vi "실습 6-2 신호시뮬레이션(이벤트).vi"() -> ()   [LabVIEW 2014]
uses:
  <vilib>/Analysis/NI_AALBase.lvlib
panel:
  in  "정지":bool
  out "웨이브폼 그래프":dbl[](graph)
  in  "열거형":enum16{"사인파", "삼각파", "사각파", "톱니파", "노이즈"}(ring)
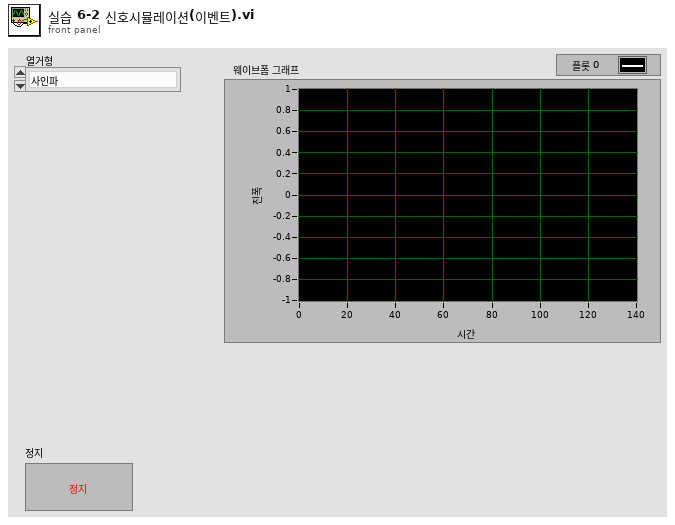
[diagram p1: front panel]
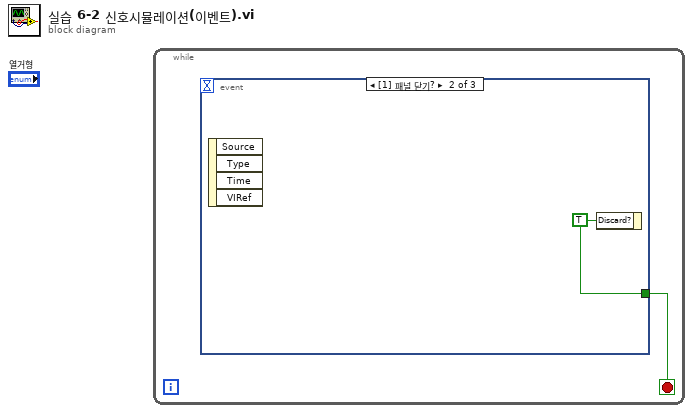
[diagram p0: block diagram]
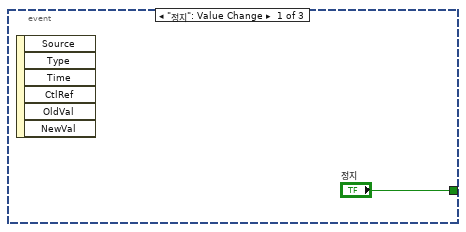
[diagram p2: hidden frame]
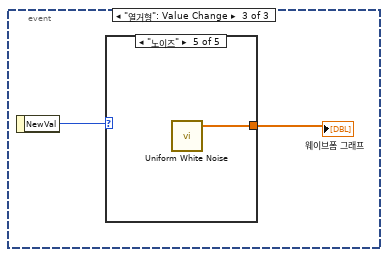
[diagram p3: hidden frame]
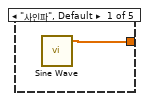
[diagram p4: hidden frame]
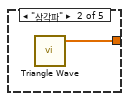
[diagram p5: hidden frame]
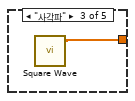
[diagram p6: hidden frame]
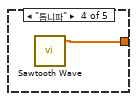
[diagram p7: hidden frame]
diagram:
  n1 = while {
    stop <- w1 stop-if-true
    n2 = event shown="[1] 패널 닫기?" {
      selector: _ -> [_ _ _]
      dyn-events: _ -> [_ _ _]
      timeout: _ -> [_ _ _]
      tunnel: ["정지" w3 _] -> w1
      event "정지": Value Change {
        n3 = event-data() -> ()  [unwired: 1 in, 6 out]
      }
      event Panel Close? {
        w3 = TRUE ("버림?")
        n4 = event-data() -> ()  [unwired: 1 in, 4 out]
        n5 = event-data("Discard?"=w3) -> ()  [unwired: 1 in, 1 out]
      }
      event "열거형": Value Change {
        n6 = event-data() -> ("NewVal"=w5:enum16{"사인파", "삼각파", "사각파", "톱니파", "노이즈"})  [unwired: 1 in]
        n7 = case shown="\"노이즈\"" w5 {
          tunnel: [w6 w7 w8 w9 w10] -> w4
          frame "사인파", Default {
            n8 = call <vilib>:"Sine Wave.vi"() -> ("sine wave"=w6:dbl[])  [unwired: 5 in, 2 out]
          }
          frame "삼각파" {
            n9 = call <vilib>:"Triangle Wave.vi"() -> ("triangle wave"=w7:dbl[])  [unwired: 5 in, 2 out]
          }
          frame "사각파" {
            n10 = call <vilib>:"Square Wave.vi"() -> ("square wave"=w8:dbl[])  [unwired: 6 in, 2 out]
          }
          frame "톱니파" {
            n11 = call <vilib>:"Sawtooth Wave.vi"() -> ("sawtooth wave"=w9:dbl[])  [unwired: 5 in, 2 out]
          }
          frame "노이즈" {
            n12 = call <vilib>:"Uniform White Noise.vi"() -> ("uniform white noise"=w10:dbl[])  [unwired: 10 in, 1 out]
          }
        }
        "웨이브폼 그래프" <- w4
      }
    }
  }
